vi "Generator&oscilloscope_save_diff_type.vi"() -> ()   [LabVIEW 2018]
uses:
  <instrlib>/LeCroy Wave Series/Public/Data/Read Single Waveform.vi
  <vilib>/Waveform/WDTFileIO.llb/ Write Waveform to File.vi
  <instrlib>/Siglent SDG X Series/Siglent SDG X Series.lvlib
  <instrlib>/LeCroy Wave Series/LeCroy Wave Series.lvlib
panel:
  out "error out 2":errorcluster
  in  "Tab Control":enum32{"Page 1", "Page 2"}(tab)
  in  "VISA Refnum in":refnum<visa-resource-name>
  in  "error in (no error)":errorcluster
  in  "Channel (1:Channel 1)":i32(ring)=1 items=["Channel 1"=1, "Channel 2"=2]
  in  "Enable Output (T: Enable)":bool=TRUE
  in  "Amplitude (1.0 Vpp)":dbl=1.0 format="%#.3f"
  in  "Frequency (1000 Hz)":dbl=1000.0 format="%#.6g"
  in  "DC Offset (0.00 V) in":dbl
  in  "Waveform Function (0: Sine) in":u16(ring) items=["Sine", "Square", "Ramp", "DC", "Pulse", "Arb"]
  in  "Phase (0.0 degrees)":dbl=0.002 min=-360.0 max=360.0 format="%#.1g"
  in  "Fall (20 ns)":dbl=2e-08 format="%#.3g"
  in  "Duty (20%)":dbl=20.0 min=0.0001 max=100.0 format="%.4g"
  in  "Delay (0.00 s)":dbl min=-1000000.0 max=1000000.0
  in  "Rise (20 ns)":dbl=2e-08 format="%#.3g"
  in  "True To \ngenerate\n pulse":bool
  out "VISA resource name out":refnum<visa-resource-name>
  out "error out":errorcluster
  in  "file path (dialog if empty)":path
  out ".not. x?":bool
  in  "stop data aquisation":bool
  out "Waveform Data":waveform(dbl)(graph)
  in  "Timeout (10000 ms)":u32=10000
  in  "Source (0: Channel 1)":u16(ring) items=["Channel 1", "Channel 2", "Channel 3", "Channel 4", "Memory 1", "Memory 2", "Memory 3", "Memory 4", "Function 1", "Function 2", "Function 3", "Function 4", "Function 5", "Function 6", "Function 7", "Function 8"]
  in  "Perform Auto Setup?":bool
  in  "Reset Scope?":bool
  in  "VISA resource name":refnum<visa-resource-name>
  out "output file refnum":refnum<file>
  out "Filename Out":path
  out "new file path (Not A Path if cancelled)":path
  out "Saving Data":bool
  # "Set PULSE parameters"
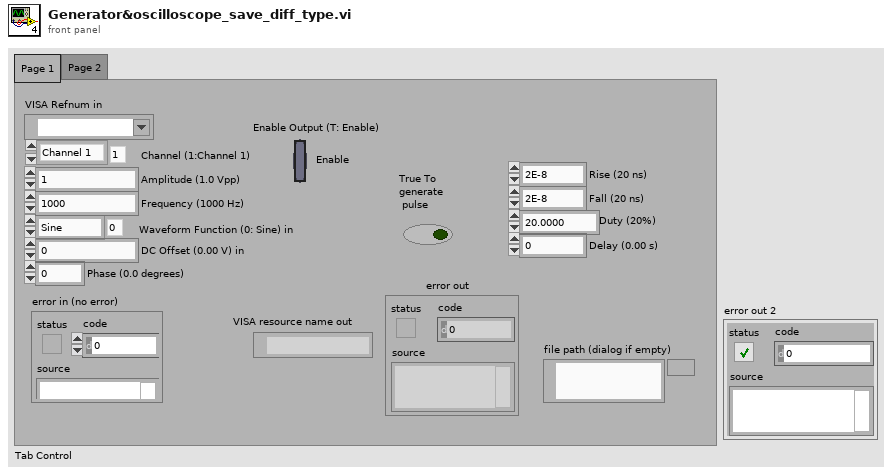
[diagram p1: front panel]
types:
  T1 = enum16{"open", "replace", "create", "open or create", "replace or create", "replace or create with confirmation"}
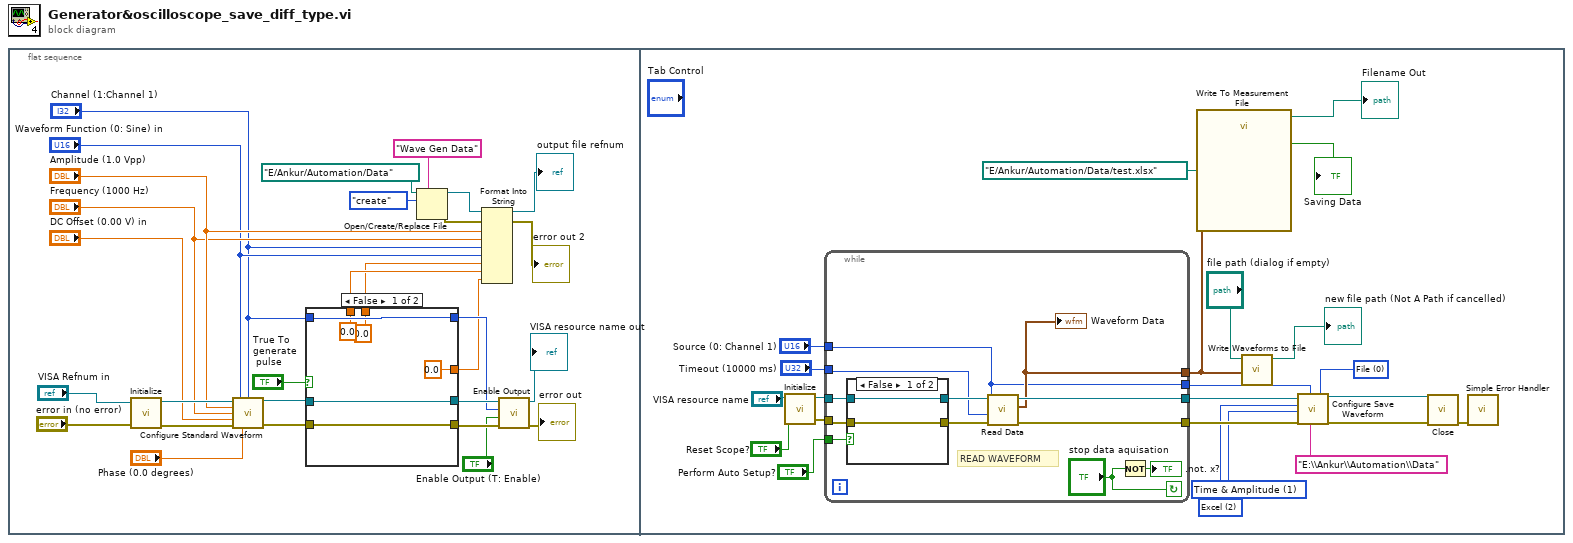
[diagram p0: block diagram]
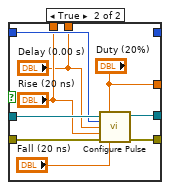
[diagram p2: hidden frame]
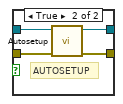
[diagram p3: hidden frame]
diagram:
  n1 = flat-sequence {
    frame #0 {
      n2 = call <instrlib>:"Initialize.vi"("error in (no error)"="error in (no error)", "VISA resource name"="VISA Refnum in") -> ("error out"=w22:errorcluster, "VISA resource name out"=w23:refnum<visa-resource-name>)  [unwired: 8 in]
      n3 = call <instrlib>:"Configure Standard Waveform.vi"("VISA resource name"=w23, "Waveform Function (0: Sine)"="Waveform Function (0: Sine) in", "Channel (1:Channel 1)"="Channel (1:Channel 1)", "Amplitude (1.0 Vpp)"="Amplitude (1.0 Vpp)", "Frequency (1000 Hz)"="Frequency (1000 Hz)", "DC Offset (0.00 V)"="DC Offset (0.00 V) in", "error in (no error)"=w22, "Phase (0.0 degrees)"="Phase (0.0 degrees)") -> ("VISA resource name out"=w18:refnum<visa-resource-name>, "error out"=w21:errorcluster)  [unwired: 6 in]
      n4 = case shown="False" "True To \ngenerate\n pulse" {
        tunnel: [w33 w41] -> w28
        tunnel: [w32 w40] -> w27
        tunnel: w18 -> [w33 w39]
        tunnel: w21 -> [w32 w38]
        tunnel: "Channel (1:Channel 1)" -> [_ w37]
        tunnel: "Channel (1:Channel 1)" -> [_ _]
        tunnel: [0.0 ("Duty (20%)") "Duty (20%)"] -> w3
        tunnel: [0.0 ("Rise (20 ns)") "Rise (20 ns)"] -> w2
        tunnel: [0.0 ("Delay (0.00 s)") "Delay (0.00 s)"] -> w1
        frame False {
        }
        frame True {
          n5 = call <instrlib>:"Configure Pulse.vi"("VISA resource name"=w39, "Duty (20%)"="Duty (20%)", "Channel (1:Channel 1)"=w37, "Delay (0.00 s)"="Delay (0.00 s)", "Rise (20 ns)"="Rise (20 ns)", "error in (no error)"=w38, "Fall (20 ns)"="Fall (20 ns)") -> ("VISA resource name out"=w41:refnum<visa-resource-name>, "error out"=w40:errorcluster)  [unwired: 7 in]
        }
      }
      n6 = Open/Create/Replace File(file path (use dialog)=path "E:/Ankur/Automation/Data" ("input file"), prompt="Wave Gen Data", operation (0:open)=T1."create") -> (refnum out=w7:refnum<file>, error out=w8:errorcluster)  [unwired: 3 in, 1 out]
      n7 = Format Into String(initial string=w7, error in=w8, "Amplitude (1.0 Vpp)", "Frequency (1000 Hz)", "Channel (1:Channel 1)", "Waveform Function (0: Sine) in", w1, w2, w3) -> (resulting string=→"output file refnum":refnum<file>, error out=→"error out 2":errorcluster)  [unwired: 1 in]
      n8 = call <instrlib>:"Enable Output.vi"("error in (no error)"=w27, "Enable Output (T: Enable)"="Enable Output (T: Enable)", "Channel (1:Channel 1)"="Channel (1:Channel 1)", "VISA resource name"=w28) -> ("error out"=→"error out":errorcluster, "VISA resource name out"=→"VISA resource name out":refnum<visa-resource-name>)  [unwired: 6 in]
    }
    frame #1 {
      w46 = u16 1 items=["Amplitude Only", "Time & Amplitude", "With Header"] ("SubFormat (1: Time & Amplitude)")
      w47 = u16 2 items=["Binary", "ASCII", "Excel", "MATLAB", "MathCad", "WaveML"] ("Format (0: Binary)")
      w48 = u16 0 items=["File", "M1", "M2", "M3", "M4"] ("Destination (0:File)")
      n9 = call <instrlib>:"Initialize.vi"("Reset? (T: Yes)"="Reset Scope?", "VISA resource name"="VISA resource name") -> ("error out"=w62:errorcluster, "VISA resource name out"=w63:refnum<visa-resource-name>)  [unwired: 8 in]
      n10 = while {
        tunnel: [w75] -> w52
        tunnel: [w74] -> w53
        tunnel: "Perform Auto Setup?" -> [w73]
        tunnel: "Source (0: Channel 1)" -> [w66]
        tunnel: w62 -> [w72]
        tunnel: w63 -> [w71]
        tunnel: "Timeout (10000 ms)" -> [w70]
        tunnel: [w67] -> w56
        tunnel: [w66] -> w49
        stop <- "stop data aquisation" continue-if-true
        # "READ WAVEFORM"
        n11 = case shown="False" w73 {
          tunnel: w72 -> [w78 w83]
          tunnel: w71 -> [w79 w82]
          tunnel: [w79 w81] -> w77
          tunnel: [w78 w80] -> w76
          frame False {
          }
          frame True {
            # "AUTOSETUP"
            n12 = call <instrlib>:"Autosetup.vi"("error in (no error)"=w83, "VISA resource name"=w82) -> ("error out"=w80:errorcluster, "VISA resource name out"=w81:refnum<visa-resource-name>)  [unwired: 8 in]
          }
        }
        n13 = call-poly <instrlib>:"Read Data.vi"("error in (no error)"=w76, "Timeout (10000 ms)"=w70, "Source (0: Channel 1)"=w66, "VISA resource name"=w77) -> ("error out"=w75:errorcluster, "Waveform Data"=w67:waveform(dbl), "VISA resource name out"=w74:refnum<visa-resource-name>)  [unwired: 5 in]
        "Waveform Data" <- w67
        n14 = Not(x="stop data aquisation") -> (.not. x?=→".not. x?":bool)
      }
      n15 = call "Write To Measurement File"("Signals"=w56, "Filename"=path "E:/Ankur/Automation/Data/test.xlsx") -> ("Filename Out"=→"Filename Out":path, "Saving Data"=→"Saving Data":bool)  [unwired: 15 in, 1 out]
      n16 = call-poly <vilib>:"Write Waveforms to File.vi"("waveform"=w56, "file path (dialog if empty)"="file path (dialog if empty)") -> ("new file path (Not A Path if cancelled)"=→"new file path (Not A Path if cancelled)":path)  [unwired: 8 in, 1 out]
      n17 = call <instrlib>:"Configure Save Waveform.vi"("VISA resource name"=w53, "Format (0: Binary)"=w47, "SubFormat (1: Time & Amplitude)"=w46, "error in (no error)"=w52, "Source (0: Channel 1)"=w49, "Save Files in Directory (D:\\Waveforms)"="E:\\Ankur\\Automation\\Data" ("Save Files in Directory (D:\\Waveforms)"), "Destination (0:File)"=w48) -> ("VISA resource name out"=w51:refnum<visa-resource-name>, "error out"=w50:errorcluster)  [unwired: 11 in]
      n18 = call <instrlib>:"Close.vi"("error in (no error)"=w50, "VISA resource name"=w51) -> ("error out"=w65:errorcluster)  [unwired: 9 in]
      n19 = call <vilib>:"Simple Error Handler.vi"("error in (no error)"=w65) -> ()  [unwired: 4 in, 5 out]
    }
  }
